vi "CleanUp.vi"(0 "object in":refnum<class "Map.lvclass">, 5 "error in (no error)":errorcluster) -> (14 "object out":refnum<class "Map.lvclass">, 19 "error out":errorcluster)   [LabVIEW 2015, in "Map.lvclass"]
doc: "Cleans up all resources used by this class."
uses:
  Map.lvclass
  Map.lvclass/Map.ctl
  Battleship_class/Battleship.lvclass
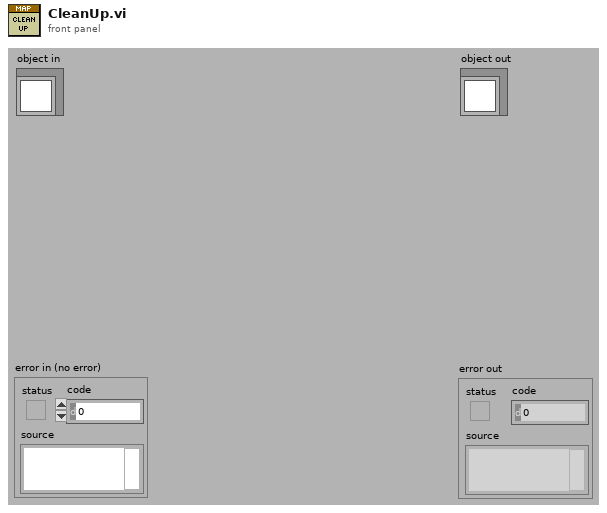
[diagram p1: front panel]
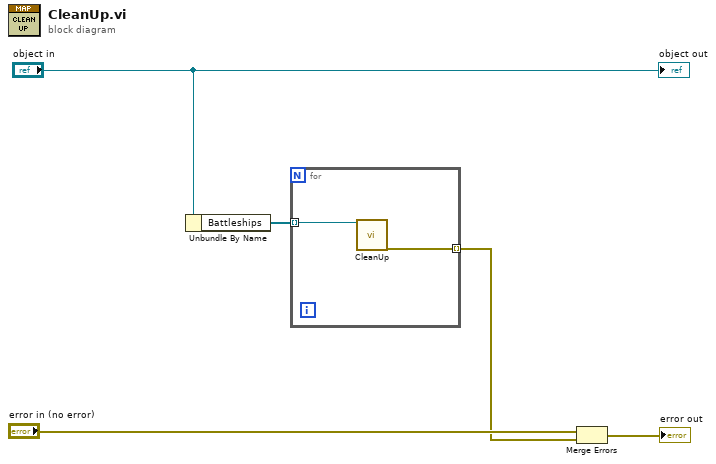
[diagram p0: block diagram]
diagram:
  n1 = Unbundle By Name("object in") -> ("Battleships"=w4:refnum<class "Battleship.lvclass">[])
  n2 = for {
    tunnel: w4 -> [w7] mode=indexing
    tunnel: [w6] -> w1 mode=indexing
    n3 = call-dynamic "CleanUp.vi"("object in"=w7) -> ("error out"=w6:errorcluster)  [unwired: 17 in, 1 out]
  }
  n4 = Merge Errors("error in (no error)", w1) -> (→"error out":errorcluster)
  "object out" <- "object in"
